vi "NextRecord.vi"(0 "reference in":refnum<class "CustomersData.lvclass">, 5 "error in (no error)":errorcluster) -> (14 "reference out":refnum<class "CustomersData.lvclass">, 19 "error out":errorcluster)   [LabVIEW 2020, in "CustomersData.lvclass"]
uses:
  CustomersData.lvclass
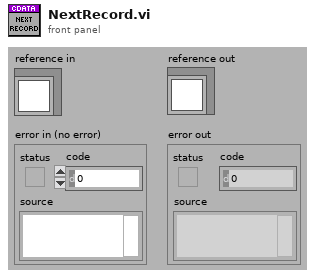
[diagram p1: front panel]
types:
  T1 = typedef "CustomersData.lvclass/ObjectAttributes.ctl" = cluster{"_customers":string[], "_current":i32}
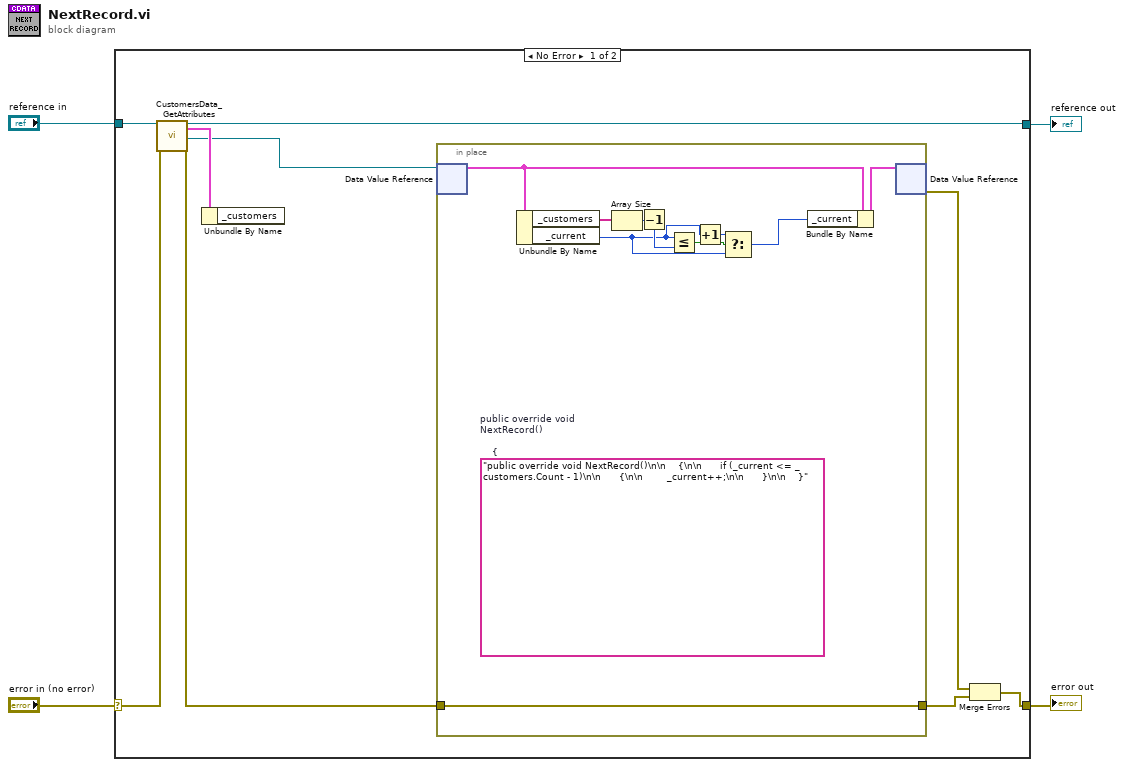
[diagram p0: block diagram]
diagram:
  n1 = case shown="No Error" "error in (no error)" {
    selector: "error in (no error)" -> [w12 w25]
    tunnel: [w9 w25] -> w3
    tunnel: [w8 w24] -> w1
    tunnel: "reference in" -> [w13 w24]
    frame No Error {
      n2 = call "CustomersData_GetAttributes.vi"("reference in"=w13, "error in (no error)"=w12) -> ("reference out"=w8:refnum<class "CustomersData.lvclass">, "Data"=w11:T1, "DataRef"=w7:refnum<data-value>, "error out"=w6:errorcluster)  [unwired: 14 in]
      n3 = Unbundle By Name(w11) -> ()  [unwired: 1 out]
      n4 = in-place {
        in-place-border: w6 -> [w22]
        in-place-border: [w22] -> w5
        (unwired) "public override void NextRecord()\n\n    {\n\n      if (_current <= _customers.Count - 1)\n\n      {\n\n        _current++;\n\n      }\n\n    }"  # public override void NextRecord()      {        if (_current <= _customers.Count - 1)        {          _current++;        }      }
        n5 = in-place-dvr #1(w7) -> (w21:T1)  [unwired: 1 out]
        n6 = Unbundle By Name(w21) -> ("_customers"=w20:string[], "_current"=w15:i32)
        n7 = Array Size(array=w20) -> (size(s)=w19:i32)
        n8 = Decrement(x=w19) -> (x-1=w18:i32)
        n9 = Less Or Equal?(x=w15, y=w18) -> (x <= y?=w17:bool)
        n10 = Increment(x=w15) -> (x+1=w16:i32)
        n11 = Select(t=w16, s=w17, f=w15) -> (s? t:f=w14:i32)
        n12 = Bundle By Name(cluster=w21, "_current"=w14) -> (w23:T1)
        n13 = in-place-dvr #1(w23) -> (w10:errorcluster)  [unwired: 1 out]
      }
      n14 = Merge Errors(w10, w5) -> (w9:errorcluster)
    }
    frame Error {
    }
  }
  "error out" <- w3
  "reference out" <- w1
